vi "Write UI Closed.vi"(10 "Subscriptions.UI Closed":refnum<class "MVC Subscription.lvclass">, 11 "Flex  Dialog (Actor) in":refnum<class "Flex Dialog (Actor).lvclass">) -> (3 "Flex  Dialog (Actor) out":refnum<class "Flex Dialog (Actor).lvclass">)   [LabVIEW 2016, in "Flex UI Dialog (Actor).lvlib" / "Flex Dialog (Actor).lvclass"]
uses:
  Flex Dialog (Actor).lvclass
  <vilib>/East West Architects/MVC Subscription/Subscription/MVC Subscription.lvclass
  Flex Dialog (Actor).lvclass/Flex Dialog (Actor).ctl
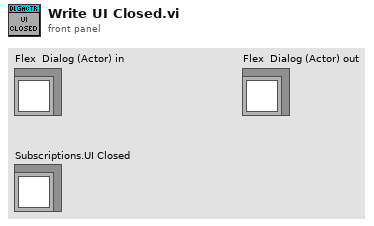
[diagram p1: front panel]
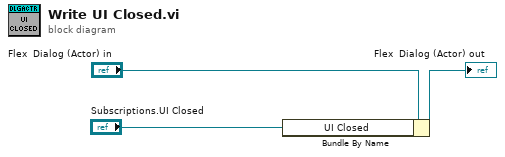
[diagram p0: block diagram]
diagram:
  n1 = Bundle By Name(cluster="Flex  Dialog (Actor) in", "UI Closed"="Subscriptions.UI Closed") -> (→"Flex  Dialog (Actor) out":refnum<class "Flex Dialog (Actor).lvclass">)
